vi "Get Elements.vi"(8 "error in (no error)":errorcluster, 11 "xwpfDocument in":refnum<class "xwpfDocument.lvclass">) -> (0 "error out":errorcluster, 2 "Elements":refnum<class "xwpfDocument.Element.lvclass">[](array[class]), 3 "xwpfDocument out":refnum<class "xwpfDocument.lvclass">)   [LabVIEW 2017, in "Word_Specific.lvlib" / "xwpfDocument.lvclass"]
uses:
  xwpfDocument.lvclass
  xwpfDocument.Element/xwpfDocument.Element.lvclass
  xwpfDocument.lvclass/xwpfDocument.ctl
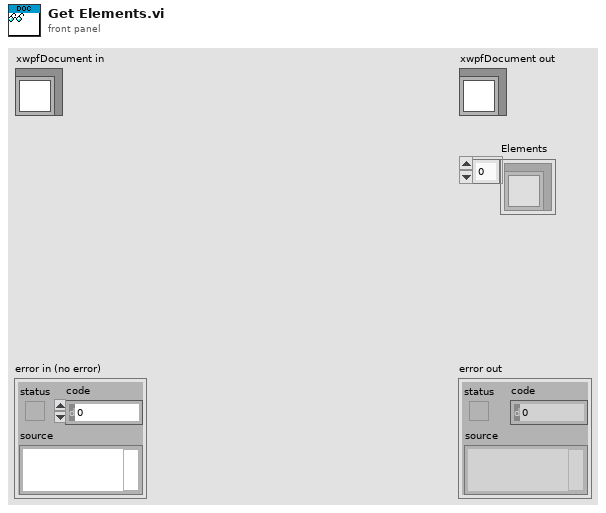
[diagram p1: front panel]
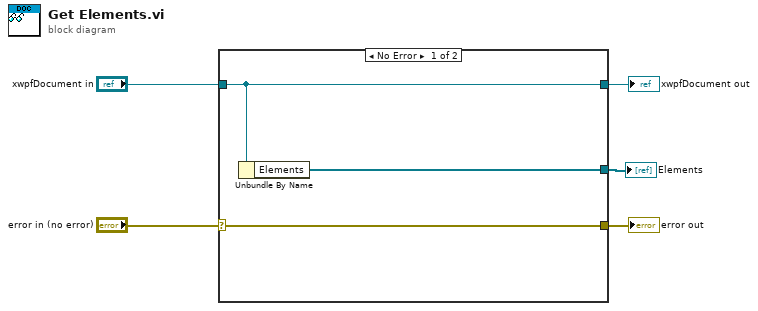
[diagram p0: block diagram]
diagram:
  n1 = case shown="No Error" "error in (no error)" {
    selector: "error in (no error)" -> [w7 w9]
    tunnel: [w7 w9] -> w4
    tunnel: [w8 w10] -> w2
    tunnel: "xwpfDocument in" -> [w8 w10]
    tunnel: [w6 _] -> w1
    frame No Error {
      n2 = Unbundle By Name(w8) -> ("Elements"=w6:refnum<class "xwpfDocument.Element.lvclass">[])
    }
    frame Error {
    }
  }
  "error out" <- w4
  "xwpfDocument out" <- w2
  "Elements" <- w1
